vi "Init File Load Dialog Data.vi"(8 "error in (no error)":errorcluster, 11 "Node Ptr":T1 format="%.0x") -> (0 "error out":errorcluster, 3 "FileDialog":T2={"File"=path "", "Group"="", "Channel"="", "DataPlugin"="", "MissingTeeth"=0.0, "ErrState"="", "File Selected"=FALSE, "Data Selection Method"=enum."Manual", "Offset"=0, "Length"=0, "DataPlugins Info"=[], "Controls"=[], "File Ref"=refnum, "Groups"=[], "Channels"=[], "Groups Refs"=[], "Channel Refs"=[], "Cancelled"=FALSE, "CycleAngle?"=FALSE, "FPGA memory size"=enum."32,768", "DAC Bits"=1, "GroupRef"=refnum, "ChanRef"=refnum, "Data"=[], "ReverseData"=FALSE} {"DAC Bits" min=1 max=16})   [LabVIEW 2011, in "Engine Sim System Explorer.lvlib"]
uses:
  Engine Sim System Explorer.lvlib
  TypeDefs/File Load Dialog.ctl
  TypeDefs/Data Replay Data Selection Method.ctl
  <vilib>/Platform/storage/utility/usiPluginInformation.ctl
  TypeDefs/AngleReference.ctl
  TypeDefs/FPGA Mem Size.ctl
  <vilib>/NI Veristand/Custom Device API/Custom Device Item Ref.ctl
  Shared/Engine Simulation Global.vi
  <vilib>/NI Veristand/Custom Device API/Get Item Property (Dependent File).vi
  <vilib>/NI Veristand/Custom Device API/Get Item Property (String).vi
  <vilib>/NI Veristand/Custom Device API/Get Item Property (Double).vi
  <vilib>/NI Veristand/Custom Device API/Get Item Property (U32).vi
  <vilib>/NI Veristand/Custom Device API/Get Item Property (Boolean).vi
  <vilib>/NI Veristand/Custom Device API/Custom Device API.lvlib
  Engine Simulation Shared.lvlib
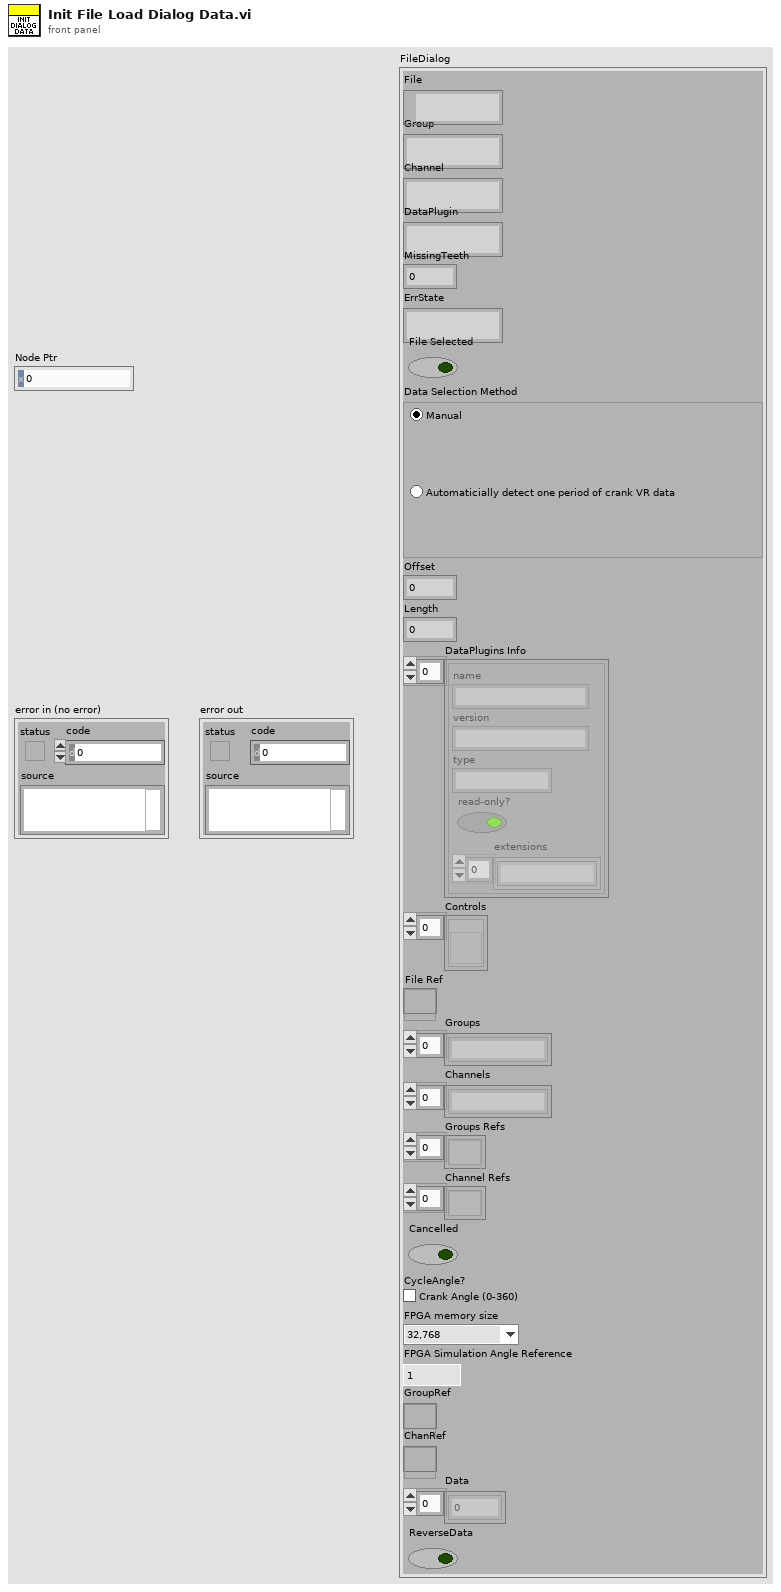
[diagram p1: front panel]
types:
  T1 = typedef "Custom Device API.lvlib/Custom Device Item Ref.ctl" = u64
  T2 = typedef "Engine Sim System Explorer.lvlib/File Load Dialog.ctl" = cluster{"File":path, "Group":string, "Channel":string, "DataPlugin":string, "MissingTeeth":dbl, "ErrState":string, "File Selected":bool, "Data Selection Method":T3, "Offset":i32, "Length":i32, "DataPlugins Info":T4[], "Controls":refnum<vi>[], "File Ref":refnum<k20>, "Groups":string[], "Channels":string[], "Groups Refs":refnum<k20>[], "Channel Refs":refnum<k20>[], "Cancelled":bool, "CycleAngle?":T5, "FPGA memory size":T6, "DAC Bits":u16, "GroupRef":refnum<k20>, "ChanRef":refnum<k20>, "Data":dbl[], "ReverseData":bool}
  T3 = typedef "Engine Sim System Explorer.lvlib/Data Replay Data Selection Method.ctl" = enum32{"Manual", "AutoVRCrank"}
  T4 = typedef "usiPluginInformation.ctl" = cluster{"name":string, "version":string, "type":string, "read-only?":bool, "extensions":string[]}
  T5 = typedef "Engine Sim System Explorer.lvlib/AngleReference.ctl" = bool
  T6 = typedef "Engine Sim System Explorer.lvlib/FPGA Mem Size.ctl" = enum16{"32,768", "16,384", "8,192", "4,096", "2,048", "1024", "512", "256", "128"}
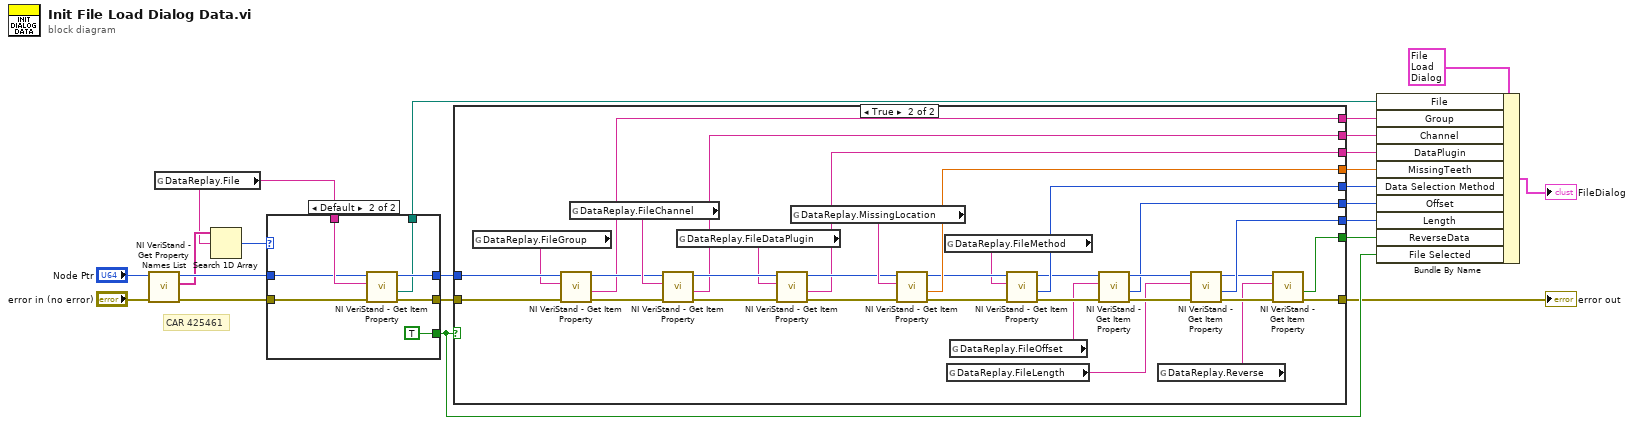
[diagram p0: block diagram]
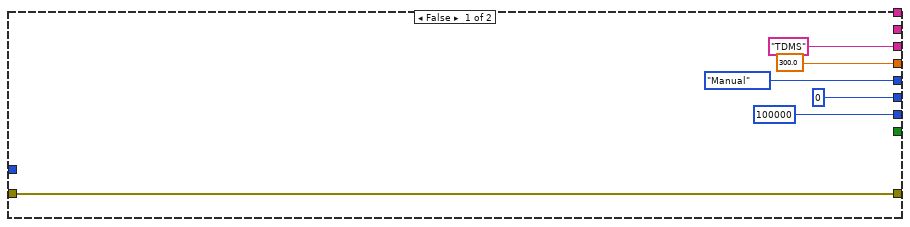
[diagram p3: hidden frame]
diagram:
  # "CAR 425461"
  n1 = call <vilib>:"NI VeriStand - Get Property Names List.vi"("error in (no error)"="error in (no error)", "Item Ref in"="Node Ptr") -> ("error out"=w7:errorcluster, "Property Names"=w4:string[], "Item Ref out"=w5:T1)  [unwired: 7 in]
  n2 = global read "Engine Simulation Global.vi" "DataReplay.File"() -> (w3:string)
  n3 = Search 1D Array(1D array=w4, element=w3) -> (index of element=w2:i32)  [unwired: 1 in]
  n4 = case shown="Default" w2 {
    tunnel: [_ TRUE] -> w22
    tunnel: [w24 w31] -> w14
    tunnel: [w23 w30] -> w13
    tunnel: [_ w29] -> w8
    tunnel: w3 -> [_ w28]
    tunnel: w7 -> [w24 w27]
    tunnel: w5 -> [w23 w26]
    frame -1 {
    }
    frame Default {
      n5 = call-poly <vilib>:"NI VeriStand - Get Item Property.vi"("error in (no error)"=w27, "Property Name"=w28, "Item Ref in"=w26) -> ("error out"=w31:errorcluster, "Path"=w29:path, "Item Ref out"=w30:T1)  [unwired: 4 in, 2 out]
    }
  }
  n6 = case shown="True" w22 {
    tunnel: w13 -> [_ w70]
    tunnel: w14 -> [w35 w69]
    tunnel: [w35 w41] -> w21
    tunnel: [_ w58] -> w16
    tunnel: [_ w57] -> w17
    tunnel: ["TDMS" ("Default Value") w56] -> w18
    tunnel: [300.0 w55] -> w19
    tunnel: [Data_Replay_Data_Selection_Method."Manual" ("Data Selection Method") w51] -> w11
    tunnel: [u32 0 ("Value") w43] -> w10
    tunnel: [u32 100000 ("Value") w42] -> w9
    tunnel: [_ w38] -> w1
    frame False {
    }
    frame True {
      n7 = global read "Engine Simulation Global.vi" "DataReplay.FileGroup"() -> (w68:string)
      n8 = call-poly <vilib>:"NI VeriStand - Get Item Property.vi"("error in (no error)"=w69, "Property Name"=w68, "Item Ref in"=w70) -> ("error out"=w65:errorcluster, "Value"=w58:string, "Item Ref out"=w66:T1)  [unwired: 5 in, 1 out]
      n9 = global read "Engine Simulation Global.vi" "DataReplay.FileChannel"() -> (w67:string)
      n10 = call-poly <vilib>:"NI VeriStand - Get Item Property.vi"("error in (no error)"=w65, "Property Name"=w67, "Item Ref in"=w66) -> ("error out"=w63:errorcluster, "Value"=w57:string, "Item Ref out"=w64:T1)  [unwired: 5 in, 1 out]
      n11 = global read "Engine Simulation Global.vi" "DataReplay.FileDataPlugin"() -> (w62:string)
      n12 = call-poly <vilib>:"NI VeriStand - Get Item Property.vi"("error in (no error)"=w63, "Property Name"=w62, "Item Ref in"=w64) -> ("error out"=w59:errorcluster, "Value"=w56:string, "Item Ref out"=w60:T1)  [unwired: 5 in, 1 out]
      n13 = global read "Engine Simulation Global.vi" "DataReplay.MissingLocation"() -> (w61:string)
      n14 = call-poly <vilib>:"NI VeriStand - Get Item Property.vi"("error in (no error)"=w59, "Property Name"=w61, "Item Ref in"=w60) -> ("error out"=w53:errorcluster, "Value"=w55:dbl, "Item Ref out"=w54:T1)  [unwired: 5 in, 1 out]
      n15 = global read "Engine Simulation Global.vi" "DataReplay.FileMethod"() -> (w52:string)
      n16 = global read "Engine Simulation Global.vi" "DataReplay.FileLength"() -> (w44:string)
      n17 = global read "Engine Simulation Global.vi" "DataReplay.FileOffset"() -> (w45:string)
      n18 = call-poly <vilib>:"NI VeriStand - Get Item Property.vi"("error in (no error)"=w53, "Property Name"=w52, "Item Ref in"=w54) -> ("error out"=w49:errorcluster, "Value"=w51:u32, "Item Ref out"=w50:T1)  [unwired: 5 in, 1 out]
      n19 = call-poly <vilib>:"NI VeriStand - Get Item Property.vi"("error in (no error)"=w49, "Property Name"=w45, "Item Ref in"=w50) -> ("error out"=w47:errorcluster, "Value"=w43:u32, "Item Ref out"=w48:T1)  [unwired: 5 in, 1 out]
      n20 = global read "Engine Simulation Global.vi" "DataReplay.Reverse"() -> (w39:string)
      n21 = call-poly <vilib>:"NI VeriStand - Get Item Property.vi"("error in (no error)"=w47, "Property Name"=w44, "Item Ref in"=w48) -> ("error out"=w46:errorcluster, "Value"=w42:u32, "Item Ref out"=w40:T1)  [unwired: 5 in, 1 out]
      n22 = call-poly <vilib>:"NI VeriStand - Get Item Property.vi"("error in (no error)"=w46, "Property Name"=w39, "Item Ref in"=w40) -> ("error out"=w41:errorcluster, "Value"=w38:bool)  [unwired: 5 in, 2 out]
    }
  }
  "error out" <- w21
  n23 = Bundle By Name(cluster=T2 {"File"=path "", "Group"="", "Channel"="", "DataPlugin"="", "MissingTeeth"=0.0, "ErrState"="", "File Selected"=FALSE, "Data Selection Method"=enum."Manual", "Offset"=0, "Length"=0, "DataPlugins Info"=[], "Controls"=[], "File Ref"=refnum, "Groups"=[], "Channels"=[], "Groups Refs"=[], "Channel Refs"=[], "Cancelled"=FALSE, "CycleAngle?"=FALSE, "FPGA memory size"=enum."32,768", "DAC Bits"=0, "GroupRef"=refnum, "ChanRef"=refnum, "Data"=[], "ReverseData"=FALSE} ("FileDialog"), "File"=w8, "Group"=w16, "Channel"=w17, "DataPlugin"=w18, "MissingTeeth"=w19, "Data Selection Method"=w11, "Offset"=w10, "Length"=w9, "ReverseData"=w1, "File Selected"=w22) -> (→"FileDialog":T2)
